vi "Screenshot.vi"(8 "error in (no error)":errorcluster caption="错误输入（无错误）") -> (0 "error out":errorcluster caption="错误输出")   [LabVIEW 2012]
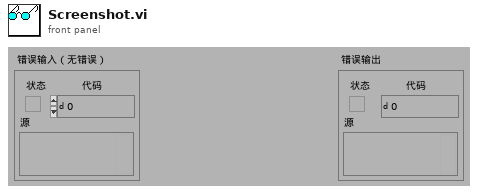
[diagram p1: front panel]
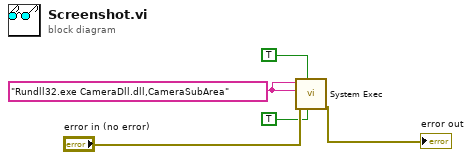
[diagram p0: block diagram]
diagram:
  w5 = "Rundll32.exe CameraDll.dll,CameraSubArea" ("standard input")
  n1 = call <vilib>:"System Exec.vi"("run minimized? (F)"=TRUE, "wait until completion? (T)"=TRUE, "error in (no error)"="error in (no error)", "standard input"=w5, "command line"=w5) -> ("error out"=→"error out":errorcluster)  [unwired: 3 in, 3 out]
